vi "to string 1.0.vi"(8 "error in (no error)":errorcluster, 10 "data in":string, 11 "Increment configuration in":refnum<class "Increment configuration.lvclass">) -> (0 "error out":errorcluster, 2 "data out":string, 3 "Increment configuration out":refnum<class "Increment configuration.lvclass">)   [LabVIEW 2015, in "Increment configuration.lvclass"]
uses:
  Increment configuration.lvclass
  Increment configuration.lvclass/Increment configuration.ctl
  <vilib>/NI/Tag Bus Module Framework/channel/TBM channel.lvclass
  <vilib>/NI/Configuration Framework/serializable configuration/NISE_CEF_serializable configuration.lvclass
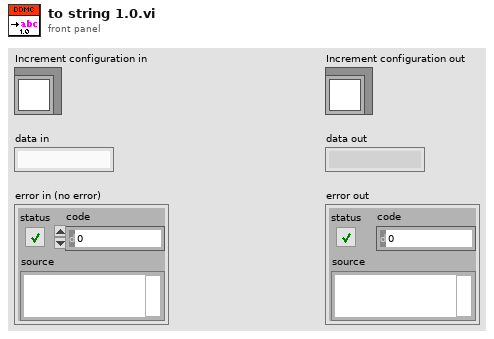
[diagram p1: front panel]
types:
  T1 = typedef "Increment configuration.lvclass/Line.ctl" = cluster{"Name":string, "channel in":refnum<class "TBM channel.lvclass">, "channel out":refnum<class "TBM channel.lvclass">}
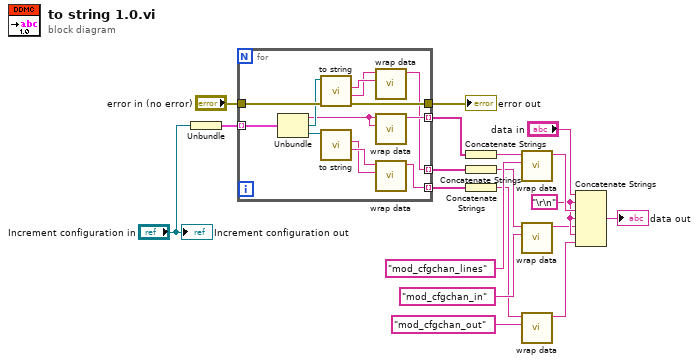
[diagram p0: block diagram]
diagram:
  w3 = "\r\n"
  n1 = Unbundle("Increment configuration in") -> (w11:T1[])
  n2 = for {
    tunnel: w11 -> [w32] mode=indexing
    tunnel: [w23] -> w12 mode=indexing
    tunnel: "error in (no error)" -> [w29]
    tunnel: [w28] -> w19
    tunnel: [w22] -> w5 mode=indexing
    tunnel: [w21] -> w4 mode=indexing
    n3 = Unbundle(w32) -> ("Name"=w20:string, "channel in"=w26:refnum<class "TBM channel.lvclass">, "channel out"=w27:refnum<class "TBM channel.lvclass">)
    n4 = call-dynamic "to string.vi"("error in"=w29, "channel in"=w26) -> ("error out"=w28:errorcluster, "channel data"=w30:string, "identifier"=w31:string)  [unwired: 6 in, 1 out]
    n5 = call-dynamic "to string.vi"("channel in"=w27) -> ("channel data"=w25:string, "identifier"=w24:string)  [unwired: 7 in, 2 out]
    n6 = call <vilib>:"wrap data.vi"("identifier"=w31, "data to wrap"=w30) -> ("wrapped data"=w22:string)  [unwired: 9 in]
    n7 = call <vilib>:"wrap data.vi"("identifier"=w20, "data to wrap"=w20) -> ("wrapped data"=w23:string)  [unwired: 9 in]
    n8 = call <vilib>:"wrap data.vi"("identifier"=w24, "data to wrap"=w25) -> ("wrapped data"=w21:string)  [unwired: 9 in]
  }
  "error out" <- w19
  n9 = Concatenate Strings(w12) -> (w13:string)
  n10 = Concatenate Strings(w5) -> (w6:string)
  n11 = Concatenate Strings(w4) -> (w7:string)
  n12 = call <vilib>:"wrap data.vi"("identifier"="mod_cfgchan_lines", "data to wrap"=w13) -> ("wrapped data"=w16:string)  [unwired: 9 in]
  n13 = call <vilib>:"wrap data.vi"("identifier"="mod_cfgchan_in", "data to wrap"=w6) -> ("wrapped data"=w2:string)  [unwired: 9 in]
  n14 = call <vilib>:"wrap data.vi"("identifier"="mod_cfgchan_out", "data to wrap"=w7) -> ("wrapped data"=w1:string)  [unwired: 9 in]
  n15 = Concatenate Strings("data in", w3, w16, w3, w2, w3, w1) -> (→"data out":string)
  "Increment configuration out" <- "Increment configuration in"
